vi "Get.vi"(11 "Boolean in":refnum<class "Boolean.lvclass">) -> (2 "Value":bool)   [LabVIEW 2020, in "Conditu2.lvlib" / "Columns.lvlib" / "Boolean.lvclass"]
uses:
  Boolean.lvclass
  Boolean.lvclass/Boolean.ctl
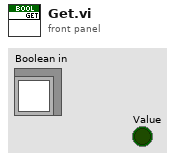
[diagram p1: front panel]
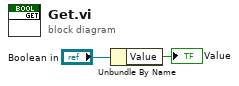
[diagram p0: block diagram]
diagram:
  n1 = Unbundle By Name("Boolean in") -> ("Value"=→"Value":bool)
